vi "New.vi"(8 "error in (no error)":errorcluster) -> (0 "error out":errorcluster, 3 "separator item out":refnum<class "separator item.lvclass">)   [LabVIEW 2009, in "separator item.lvclass"]
uses:
  separator item.lvclass
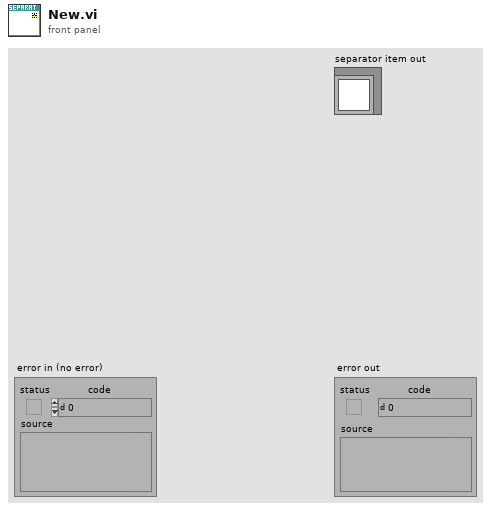
[diagram p1: front panel]
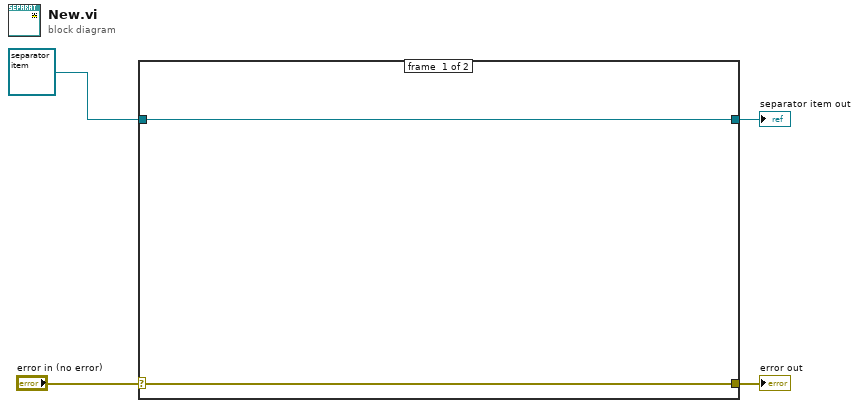
[diagram p0: block diagram]
diagram:
  n1 = case shown="No Error" "error in (no error)" {
    selector: "error in (no error)" -> [w5 w8]
    tunnel: [w5 w8] -> w1
    tunnel: [w6 w7] -> w3
    tunnel: refnum<class "separator item.lvclass"> refnum ("seperator item in") -> [w6 w7]
    frame #0 {
    }
    frame #1 {
    }
  }
  "separator item out" <- w3
  "error out" <- w1
